vi "Motor controller.vi"() -> ()   [LabVIEW 2015]
uses:
  Motor controller/Signaller/Signaller.lvclass
  Motor controller/Motor/Motor.lvclass
  Motor controller/Automatic mode/Automatic Mode.lvclass
  Motor controller/Motor/AlphaStep One/AlphaStep One.lvclass
  Motor controller/Motor/Dummy Motor/Dummy Motor.lvclass
panel:
  in  "Home frequency 2":cluster{"Positive":dbl, "Negative":dbl}={"Positive"=140.18, "Negative"=140.45} {"Negative" format="%.3g"; "Positive" format="%.3g"}
  in  "Home frequency":cluster{"Positive":dbl, "Negative":dbl}={"Positive"=140.18, "Negative"=140.45} {"Negative" format="%.3g"; "Positive" format="%.3g"}
  in  "Negative seek bounds":cluster{"Minimum":dbl, "Maximum":dbl}={"Minimum"=140.35, "Maximum"=140.65} {"Maximum" format="%.3g"; "Minimum" format="%.3g"}
  in  "Positive seek bounds":cluster{"Minimum":dbl, "Maximum":dbl}={"Minimum"=140.0, "Maximum"=140.3} {"Maximum" format="%.3g"; "Minimum" format="%.3g"}
  in  "Debug mode":bool
  out "Grapher VI":refnum<vi>
  out "Simulation VI":refnum<vi>
  in  "0.01 GHz/step":bool
  in  "0.05 GHz/step":bool
  in  "0.03 GHz/step":bool
  in  "Reset everything":bool
  in  "Make up fit parameters":bool
  in  "Automatic velocity (rev/sec)":dbl=0.1 min=0.0 max=1.0
  in  "Reseek":bool
  in  "Automatic step size (rev)":dbl=0.01 min=0.0 max=1.0
  in  "Step size (GHz)":dbl min=0.0 max=1.0 step=0.001 format="%.3g"
  in  "Goto frequency":bool
  in  "Frequency to seek (GHz)":dbl format="%.3g"
  in  "Stop motor":bool
  in  "Move up":bool
  in  "Move down":bool
  in  "Velocity (rev/sec)":dbl min=0.0 max=1.0 step=0.001
  in  "Step size (rev)":dbl=0.01 min=0.0 max=5.0 step=0.001 format="%.3g"
  in  "Restore configuration from file":bool
  in  "Save configuration to file":bool
  in  "Refine fit parameters":bool
  out "Fit parameters":cluster{"Slope":dbl, "Intercept":dbl}
  in  "Calculate fit parameters":bool
  in  "Read position 2":bool
  in  "Read position 1":bool
  out "Position 2":dbl
  in  "Frequency 2":dbl=140.4 min=0.0 step=0.001 format="%.3g"
  out "Position 1":dbl
  in  "Frequency 1":dbl=140.0 min=0.0 step=0.001 format="%.3g"
  in  "Seek positive polarization":bool=TRUE
  in  "Launch simulation":bool
  out "Polarization":dbl
  out "Eventnum":i64
  out "Samples taken":i32
  out "Rate":dbl
  in  "Data input file":path
  in  "Automatic mode on/off":bool
  in  "Stop communication":bool
  in  "COM Port":refnum<visa-resource-name>
  out "Alarm":bool
  out "Alarm code":i32 format="0x%02x"
  out "Frequency (calculated, GHz)":dbl format="%.3g"
  out "Motor position (rev)":dbl format="%.3g"
  out "Motor time (sec)":dbl
  # "Advanced configuration"
  # "Step size presets"
  # "Manual motor control"
  # "Configuration backup/restore"
  # "The settings which are backed up by this method are: COM port, step size, frequency to seek, fit slope, fit intercept, automatic step size, automatic velocity, and data input file."
  # "Frequency calibration"
  # "Automatic control"
  # "Communication setup"
  # "Please wait after stopping the VI; it can take some time to shut down all the stuff running in the background, so please be patient."
  # "Motor alarm (error)"
  # "See motor manual, section \"Troubleshooting\" for explanation of alarm codes; fix the problem first and then restart this VI"
  # "Motor information"
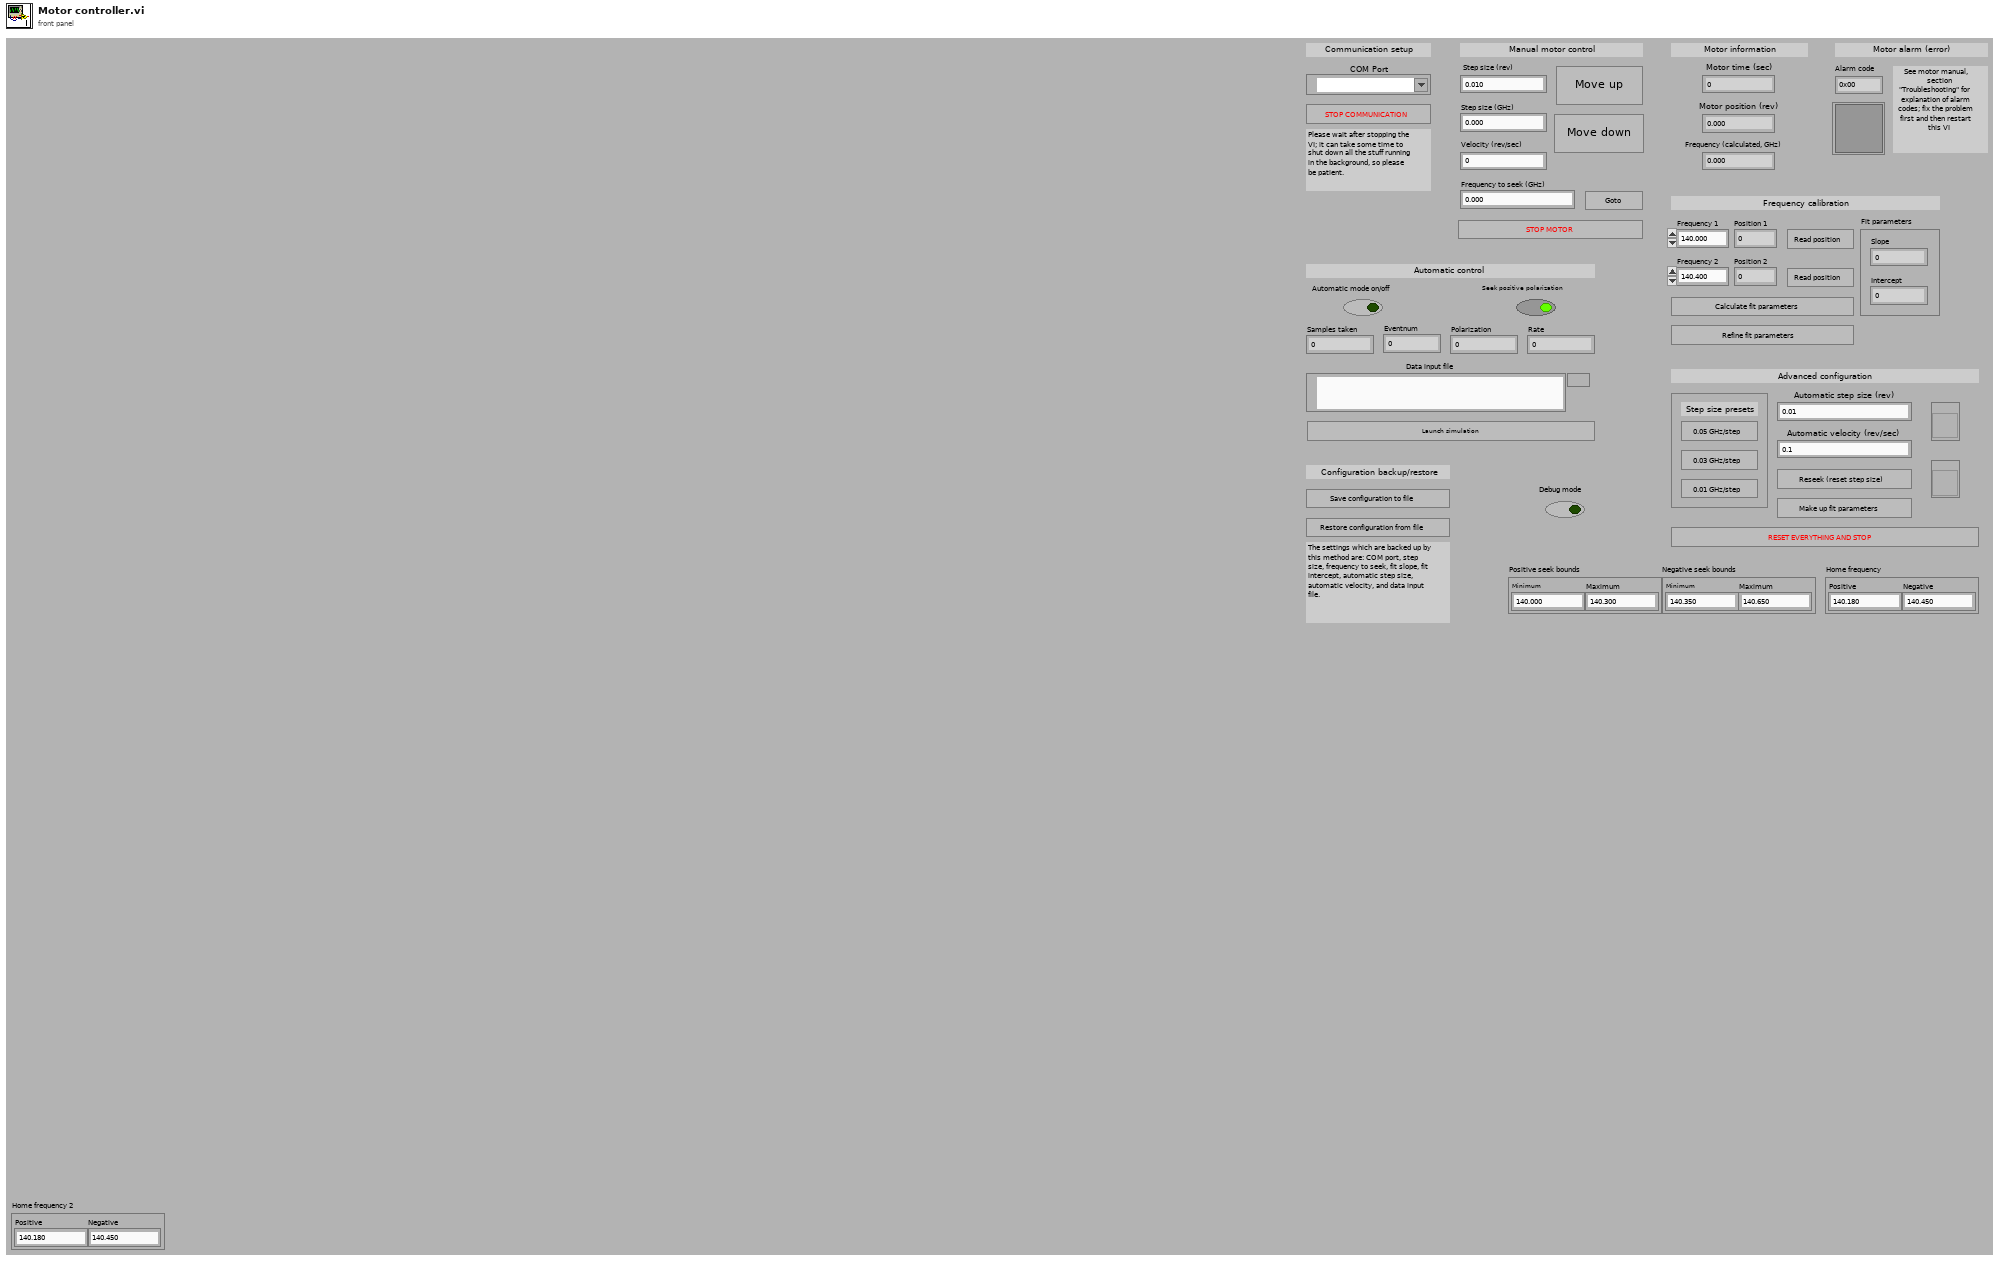
[diagram p1: front panel]
types:
  T1 = enum8{"Enabled", "Disabled", "Disabled and Grayed Out"}
  T2 = enum16{"open", "replace", "create", "open or create", "replace or create", "replace or create with confirmation"}
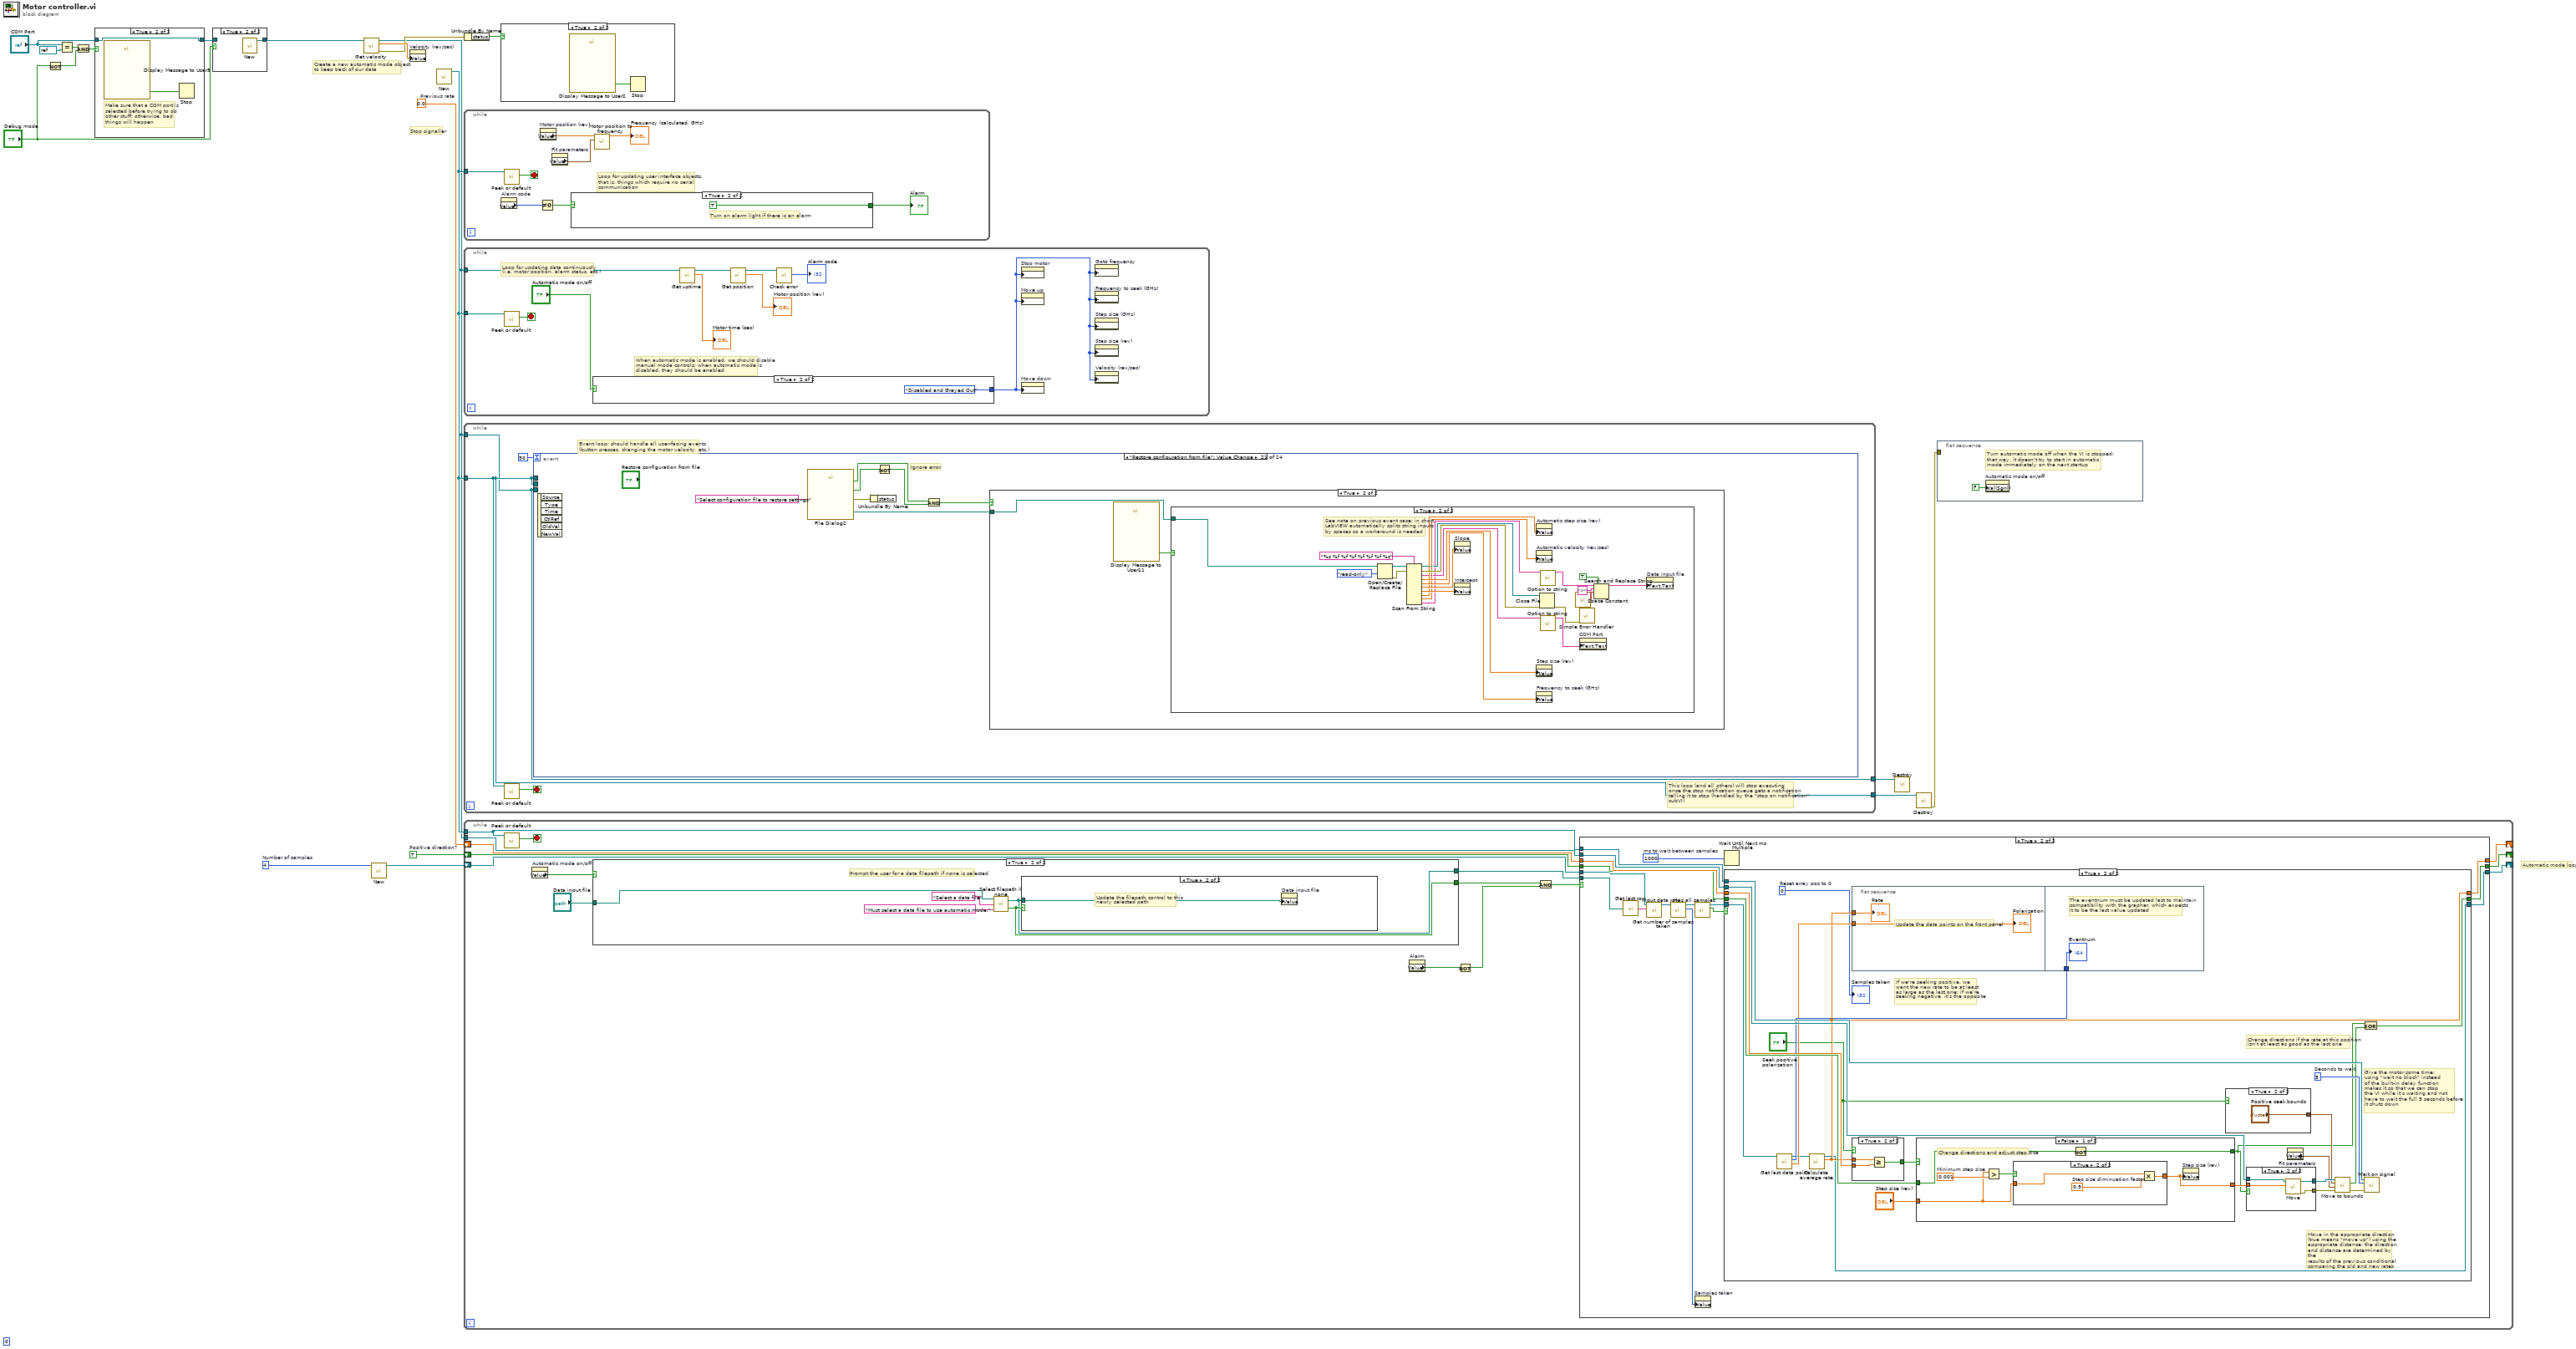
[diagram p0: block diagram]
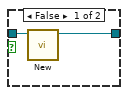
[diagram p2: hidden frame]
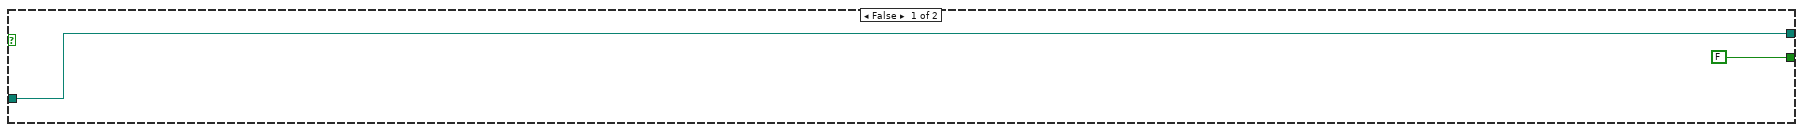
[diagram p5: hidden frame]
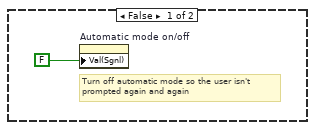
[diagram p6: hidden frame]
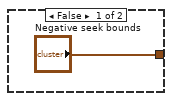
[diagram p9: hidden frame]
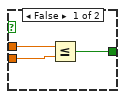
[diagram p10: hidden frame]
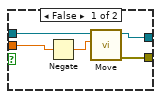
[diagram p11: hidden frame]
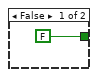
[diagram p14: hidden frame]
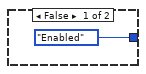
[diagram p15: hidden frame]
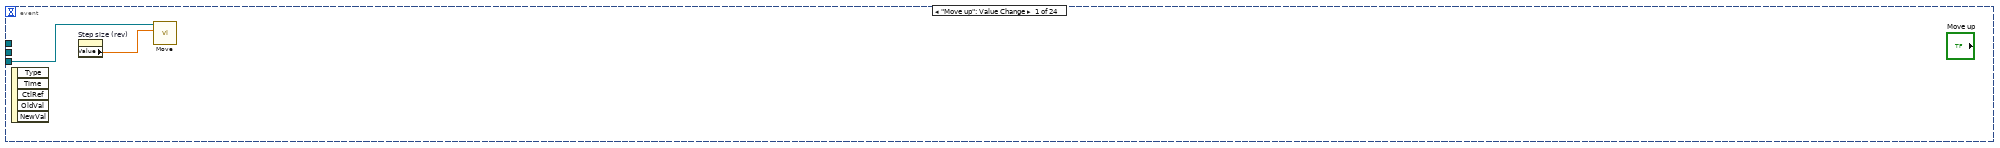
[diagram p16: hidden frame]
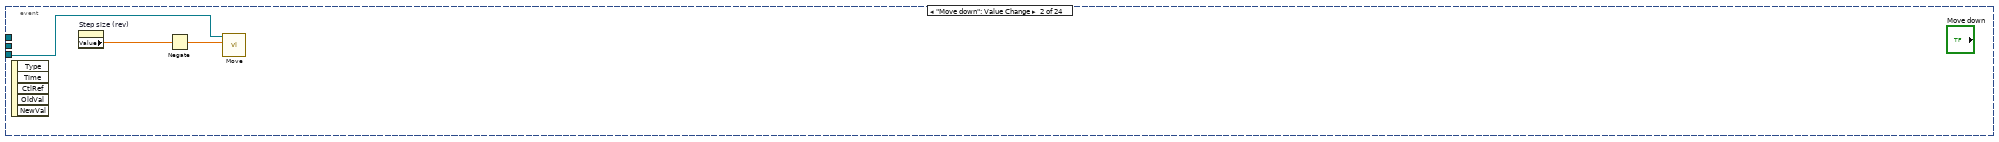
[diagram p17: hidden frame]
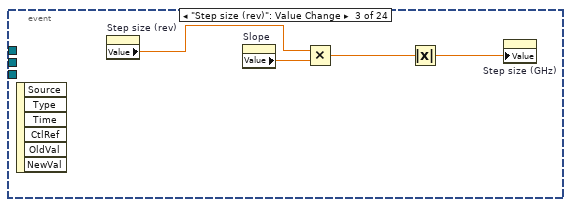
[diagram p18: hidden frame]
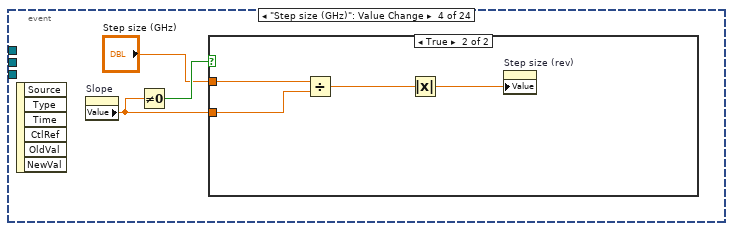
[diagram p19: hidden frame]
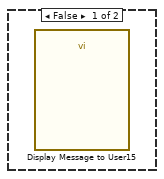
[diagram p20: hidden frame]
diagram:
  w14 = 4  # Number of samples
  w18 = TRUE  # Positive direction?
  w19 = 0.0  # Previous rate
  (unwired) i64 0
  # "Stop signaller"
  # "Create a new automatic mode object\nto keep track of our data"
  # "Automatic mode loop"
  n1 = Not(x="Debug mode") -> (.not. x?=w9:bool)
  n2 = Equal?(x="COM Port", y=refnum<visa-resource-name> refnum) -> (x = y?=w10:bool)
  n3 = And(x=w10, y=w9) -> (x .and. y?=w11:bool)
  n4 = case shown="True" w11 {
    tunnel: "COM Port" -> [w21 w22]
    tunnel: [w21 w22] -> w7
    frame False {
    }
    frame True {
      # "Make sure that a COM port is\nselected before trying to do\nother stuff; otherwise, bad\nthings will happen"
      n5 = call "Display Message to User5"() -> ("Got it, thanks"=w23:bool)  [unwired: 10 in, 1 out]
      n6 = Stop(stop? (T)=w23) -> ()
    }
  }
  n7 = case shown="True" "Debug mode" {
    tunnel: w7 -> [w25 _]
    tunnel: [w24 w26] -> w6
    frame False {
      n8 = call "New.vi"("VISA resource name"=w25) -> ("AlphaStep One out"=w24:refnum<class "AlphaStep One.lvclass">)  [unwired: 9 in, 1 out]
    }
    frame True {
      n9 = call "New.vi"() -> ("Dummy Motor out"=w26:refnum<class "Dummy Motor.lvclass">)  [unwired: 10 in, 1 out]
    }
  }
  n10 = call-dynamic "Get velocity.vi"("Motor in"=w6) -> ("error out"=w4:errorcluster, "Velocity (rev/sec)"=w5:dbl, "Motor out"=w3:refnum<class "Motor.lvclass">)  [unwired: 8 in]
  n11 = call "New.vi"("Number of samples (4)"=w14) -> ("Automatic Mode out"=w13:refnum<class "Automatic Mode.lvclass">)  [unwired: 9 in, 1 out]
  n12 = property on="Velocity (rev/sec)" class="DigNum (strict)"("Value"=w5) -> ()  [unwired: 2 in, 2 out]
  n13 = call "New.vi"() -> ("Signaller out"=w12:refnum<class "Signaller.lvclass">)  [unwired: 11 in]
  n14 = Unbundle By Name(w4) -> ("status"=w8:bool)
  n15 = while {
    tunnel: w12 -> [w30]
    stop <- w29 stop-if-true
    # "Loop for updating user interface objects,\nthat is, things which require no serial\ncommunication"
    n16 = property on="Alarm code" class="DigNum (strict)"() -> ("Value"=w28:i32)  [unwired: 2 in, 2 out]
    n17 = call "Peek or default.vi"("Signaller in"=w30) -> ("Has signal?"=w29:bool)  [unwired: 8 in, 2 out]
    n18 = property on="Motor position (rev)" class="DigNum (strict)"() -> ("Value"=w32:dbl)  [unwired: 2 in, 2 out]
    n19 = Not Equal To 0?(x=w28) -> (x != 0?=w27:bool)
    n20 = property on="Fit parameters" class="Clust (strict)"() -> ("Value"=w33:cluster{"Slope":dbl, "Intercept":dbl})  [unwired: 2 in, 2 out]
    n21 = case shown="True" w27 {
      tunnel: [FALSE TRUE] -> w34
      frame False {
      }
      frame True {
        # "Turn on alarm light if there is an alarm"
      }
    }
    "Alarm" <- w34
    n22 = call "Motor position to frequency.vi"("Fit parameters"=w33, "Motor position"=w32) -> ("Frequency"=→"Frequency (calculated, GHz)":dbl)  [unwired: 9 in]
  }
  n23 = while {
    tunnel: w3 -> [w42]
    tunnel: w12 -> [w45]
    stop <- w44 stop-if-true
    # "Loop for updating data continuously\n(i.e. motor position, alarm status, etc.)"
    # "When automatic mode is enabled, we should disable\nmanual mode controls; when automatic mode is\ndisabled, they should be enabled"
    n24 = call "Peek or default.vi"("Signaller in"=w45) -> ("Has signal?"=w44:bool)  [unwired: 8 in, 2 out]
    n25 = case shown="True" "Automatic mode on/off" {
      tunnel: [T1."Enabled" ("Disabled") T1."Disabled and Grayed Out" ("Disabled")] -> w43
      frame False {
      }
      frame True {
      }
    }
    n26 = call-dynamic "Get uptime.vi"("Motor in"=w42) -> ("Uptime (sec)"=→"Motor time (sec)":dbl, "Motor out"=w41:refnum<class "Motor.lvclass">)  [unwired: 8 in, 1 out]
    n27 = call-dynamic "Get position.vi"("Motor in"=w41) -> ("Position (rev)"=→"Motor position (rev)":dbl, "Motor out"=w38:refnum<class "Motor.lvclass">)  [unwired: 8 in, 1 out]
    n28 = call-dynamic "Check error.vi"("Motor in"=w38) -> ("Error code"=→"Alarm code":i32)  [unwired: 8 in, 2 out]
    n29 = property on="Stop motor" class="Bool"("DisabledEnum"=w43) -> ()  [unwired: 2 in, 2 out]
    n30 = property on="Move up" class="Bool"("DisabledEnum"=w43) -> ()  [unwired: 2 in, 2 out]
    n31 = property on="Move down" class="Bool"("DisabledEnum"=w43) -> ()  [unwired: 2 in, 2 out]
    n32 = property on="Goto frequency" class="Bool"("DisabledEnum"=w43) -> ()  [unwired: 2 in, 2 out]
    n33 = property on="Frequency to seek (GHz)" class="DigNum (strict)"("DisabledEnum"=w43) -> ()  [unwired: 2 in, 2 out]
    n34 = property on="Step size (GHz)" class="DigNum (strict)"("DisabledEnum"=w43) -> ()  [unwired: 2 in, 2 out]
    n35 = property on="Step size (rev)" class="DigNum (strict)"("DisabledEnum"=w43) -> ()  [unwired: 2 in, 2 out]
    n36 = property on="Velocity (rev/sec)" class="DigNum (strict)"("DisabledEnum"=w43) -> ()  [unwired: 2 in, 2 out]
  }
  n37 = while {
    tunnel: w3 -> [w49]
    tunnel: w12 -> [w50]
    tunnel: [w50] -> w20
    tunnel: [w49] -> w1
    stop <- w52 stop-if-true
    # "This loop (and all others) will stop executing\nonce the stop notification queue gets a notification\ntelling it to stop (handled by the \"stop on notification\"\nsubVI)"
    # "Event loop; should handle all user-facing events\n(button presses, changing the motor velocity, etc.)"
    n38 = call "Peek or default.vi"("Signaller in"=w50) -> ("Has signal?"=w52:bool)  [unwired: 8 in, 2 out]
    n39 = event shown="[20] \"Restore configuration from file\": Value Change" {
      selector: _ -> [_ _ _ _ _ _ _ _ _ _ _ _ _ _ _ _ _ _ _ _ _ _ _ _]
      dyn-events: _ -> [_ _ _ _ _ _ _ _ _ _ _ _ _ _ _ _ _ _ _ _ _ _ _ _]
      timeout: 50 -> [_ _ _ _ _ _ _ _ _ _ _ _ _ _ _ _ _ _ _ _ _ _ _ _]
      tunnel: w49 -> [w53 w55 _ _ w70 w72 w92 _ _ _ _ _ _ w173 w204 _ _ _ _ _ _ _ w313 _]
      tunnel: w50 -> [_ _ _ _ _ _ _ _ _ _ _ w153 _ _ _ _ _ _ _ _ _ w308 w316 _]
      tunnel: w50 -> [_ _ _ _ _ _ _ _ _ _ _ _ _ w174 _ _ _ _ _ _ _ _ _ _]
      event "Move up": Value Change {
        n40 = event-data() -> ()  [unwired: 1 in, 5 out]
        n41 = property on="Step size (rev)" class="DigNum (strict)"() -> ("Value"=w54:dbl)  [unwired: 2 in, 2 out]
        n42 = call-dynamic "Move.vi"("Amount (rev)"=w54, "Motor in"=w53) -> ()  [unwired: 8 in, 2 out]
      }
      event "Move down": Value Change {
        n43 = event-data() -> ()  [unwired: 1 in, 5 out]
        n44 = property on="Step size (rev)" class="DigNum (strict)"() -> ("Value"=w57:dbl)  [unwired: 2 in, 2 out]
        n45 = Negate(x=w57) -> (-x=w56:dbl)
        n46 = call-dynamic "Move.vi"("Amount (rev)"=w56, "Motor in"=w55) -> ()  [unwired: 8 in, 2 out]
      }
      event "Step size (rev)": Value Change {
        n47 = event-data() -> ()  [unwired: 1 in, 6 out]
        n48 = property on="Step size (rev)" class="DigNum (strict)"() -> ("Value"=w61:dbl)  [unwired: 2 in, 2 out]
        n49 = property on="Slope" class="DigNum (strict)"() -> ("Value"=w60:dbl)  [unwired: 2 in, 2 out]
        n50 = Multiply(x=w61, y=w60) -> (x*y=w59:dbl)
        n51 = Absolute Value(x=w59) -> (abs(x)=w58:dbl)
        n52 = property on="Step size (GHz)" class="DigNum (strict)"("Value"=w58) -> ()  [unwired: 2 in, 2 out]
      }
      event "Step size (GHz)": Value Change {
        n53 = event-data() -> ()  [unwired: 1 in, 6 out]
        n54 = property on="Slope" class="DigNum (strict)"() -> ("Value"=w62:dbl)  [unwired: 2 in, 2 out]
        n55 = Not Equal To 0?(x=w62) -> (x != 0?=w64:bool)
        n56 = case shown="True" w64 {
          tunnel: "Step size (GHz)" -> [_ w68]
          tunnel: w62 -> [_ w67]
          frame False {
            n57 = call "Display Message to User15"() -> ()  [unwired: 10 in, 2 out]
          }
          frame True {
            n58 = Divide(x=w68, y=w67) -> (x/y=w66:dbl)
            n59 = Absolute Value(x=w66) -> (abs(x)=w65:dbl)
            n60 = property on="Step size (rev)" class="DigNum (strict)"("Value"=w65) -> ()  [unwired: 2 in, 2 out]
          }
        }
      }
      event "Velocity (rev/sec)": Value Change {
        n61 = event-data() -> ()  [unwired: 1 in, 5 out]
        n62 = call-dynamic "Set velocity.vi"("Velocity (rev/sec)"="Velocity (rev/sec)", "Motor in"=w70) -> ()  [unwired: 8 in, 2 out]
      }
      event "Goto frequency": Value Change {
        n63 = event-data() -> ()  [unwired: 1 in, 5 out]
        n64 = property on="Fit parameters" class="Clust (strict)"() -> ("Value"=w71:cluster{"Slope":dbl, "Intercept":dbl})  [unwired: 2 in, 2 out]
        n65 = Unbundle By Name(w71) -> ("Slope"=w73:dbl)
        n66 = Equal To 0?(x=w73) -> (x = 0?=w74:bool)
        n67 = case shown="False" w74 {
          tunnel: w72 -> [w82 _]
          tunnel: w71 -> [w75 _]
          frame False {
            # "Calculate corresponding motor position and go there"
            n68 = call "Frequency to motor position.vi"("Fit parameters"=w75, "Frequency"="Frequency to seek (GHz)") -> ("Motor position"=w84:dbl)  [unwired: 9 in]
            n69 = property on="Motor position (rev)" class="DigNum (strict)"() -> ("Value"=w83:dbl)  [unwired: 2 in, 2 out]
            n70 = Subtract(x=w84, y=w83) -> (x-y=w80:dbl)
            n71 = Absolute Value(x=w80) -> (abs(x)=w79:dbl)
            n72 = Less?(x=w79, y=1.0) -> (x < y?=w76:bool)
            n73 = case shown="False" w76 {
              selector: w76 -> [_ w89]
              tunnel: [w85 w89] -> w77
              frame False {
                n74 = Two Button Dialog(message="The frequency you are attempting to go to is very far from the current position; you may run into problems. Are you sure you want to continue?", 1:"No" ("F button name (\"Cancel\")"), 2:"Yes" ("T button name (\"OK\")")) -> (T button?=w85:bool)
              }
              frame True {
              }
            }
            n75 = case shown="True" w77 {
              tunnel: w82 -> [_ w90]
              tunnel: w80 -> [_ w91]
              frame False {
              }
              frame True {
                n76 = call-dynamic "Move.vi"("Amount (rev)"=w91, "Motor in"=w90) -> ()  [unwired: 8 in, 2 out]
              }
            }
          }
          frame True {
            n77 = call "Display Message to User"() -> ()  [unwired: 10 in, 2 out]
          }
        }
      }
      event "Stop motor": Value Change {
        n78 = event-data() -> ()  [unwired: 1 in, 5 out]
        n79 = call-dynamic "Stop.vi"("Motor in"=w92) -> ()  [unwired: 9 in, 2 out]
      }
      event "Read position 1": Value Change {
        n80 = event-data() -> ()  [unwired: 1 in, 5 out]
        n81 = property on="Motor position (rev)" class="DigNum (strict)"() -> ("Value"=→"Position 1":dbl)  [unwired: 2 in, 2 out]
      }
      event "Read position 2": Value Change {
        n82 = event-data() -> ()  [unwired: 1 in, 5 out]
        n83 = property on="Motor position (rev)" class="DigNum (strict)"() -> ("Value"=→"Position 2":dbl)  [unwired: 2 in, 2 out]
      }
      event "Calculate fit parameters": Value Change {
        n84 = event-data() -> ()  [unwired: 1 in, 5 out]
        n85 = property on="Position 1" class="DigNum (strict)"() -> ("Value"=w99:dbl)  [unwired: 2 in, 2 out]
        n86 = property on="Position 2" class="DigNum (strict)"() -> ("Value"=w98:dbl)  [unwired: 2 in, 2 out]
        n87 = property on="Calculate fit parameters" class="Bool (strict)"("Value"=FALSE ("Calculate fit parameters")) -> ()  [unwired: 2 in, 2 out]
        n88 = Equal?(x=w99, y=w98) -> (x = y?=w101:bool)
        n89 = Equal?(x="Frequency 1", y="Frequency 2") -> (x = y?=w100:bool)
        n90 = Or(x=w101, y=w100) -> (x .or. y?=w95:bool)
        n91 = case shown="False" w95 {
          tunnel: w99 -> [w110 _]
          tunnel: w98 -> [w109 _]
          tunnel: "Frequency 1" -> [w108 _]
          tunnel: "Frequency 2" -> [w107 _]
          frame False {
            # "Calculate slope and intercept"
            # "The automatic step size should be around 0.02GHz\ninitially, to get a good seek"
            n92 = call "Calculate fit parameters.vi"("Frequency 2"=w107, "Frequency 1"=w108, "Position 2"=w109, "Position 1"=w110) -> ("Intercept"=w111:dbl, "Slope"=w105:dbl)
            n93 = property on="Fit parameters" class="Clust (strict)"() -> ("Value"=w113:cluster{"Slope":dbl, "Intercept":dbl})  [unwired: 2 in, 2 out]
            n94 = Divide(x=0.02, y=w105) -> (x/y=w104:dbl)
            n95 = Bundle By Name(cluster=w113, "Slope"=w105, "Intercept"=w111) -> (→"Fit parameters":cluster{"Slope":dbl, "Intercept":dbl})
            n96 = Absolute Value(x=w104) -> (abs(x)=w103:dbl)
            n97 = property on="Automatic step size (rev)" class="DigNum (strict)"("Value"=w103) -> ()  [unwired: 2 in, 2 out]
          }
          frame True {
            # "Warn the user about trying to calculate/refine\nfit parameters with invalid inputs (fit function\nMUST be bijective; i.e. slope must not be 0\nor infinity)"
            n98 = call "Display Message to User6"() -> ()  [unwired: 10 in, 2 out]
          }
        }
      }
      event "Refine fit parameters": Value Change {
        n99 = event-data() -> ()  [unwired: 1 in, 6 out]
        n100 = property on="Fit parameters" class="Clust (strict)"() -> ("Value"=w119:cluster{"Slope":dbl, "Intercept":dbl})  [unwired: 2 in, 2 out]
        n101 = Unbundle By Name(w119) -> ("Slope"=w115:dbl, "Intercept"=w114:dbl)
        n102 = Equal To 0?(x=w115) -> (x = 0?=w117:bool)
        n103 = Equal To 0?(x=w114) -> (x = 0?=w116:bool)
        n104 = And(x=w116, y=w117) -> (x .and. y?=w118:bool)
        n105 = property on="Frequency 1" class="DigNum (strict)"() -> ("Value"=w123:dbl)  [unwired: 2 in, 2 out]
        n106 = property on="Frequency 2" class="DigNum (strict)"() -> ("Value"=w122:dbl)  [unwired: 2 in, 2 out]
        n107 = property on="Position 1" class="DigNum (strict)"() -> ("Value"=w121:dbl)  [unwired: 2 in, 2 out]
        n108 = property on="Position 2" class="DigNum (strict)"() -> ("Value"=w120:dbl)  [unwired: 2 in, 2 out]
        n109 = case shown="False" w118 {
          tunnel: w123 -> [w125 _]
          tunnel: w122 -> [w124 _]
          tunnel: w121 -> [w130 _]
          tunnel: w120 -> [w129 _]
          tunnel: w115 -> [w133 _]
          tunnel: w114 -> [w132 _]
          tunnel: w119 -> [w131 _]
          frame False {
            n110 = Equal?(x=w130, y=w129) -> (x = y?=w128:bool)
            n111 = Equal?(x=w125, y=w124) -> (x = y?=w127:bool)
            n112 = Or(x=w128, y=w127) -> (x .or. y?=w126:bool)
            n113 = case shown="False" w126 {
              tunnel: w125 -> [w152 _]
              tunnel: w124 -> [w151 _]
              tunnel: w130 -> [w150 _]
              tunnel: w129 -> [w149 _]
              tunnel: w133 -> [w147 _]
              tunnel: w132 -> [w145 _]
              tunnel: w131 -> [w139 _]
              frame False {
                # "Update automatic step size as well,\nas with the \"calculate fit parameters\"\naction"
                # "Average new slope and intercept with\nold ones, to get better approximation"
                n114 = call "Calculate fit parameters.vi"("Frequency 2"=w151, "Frequency 1"=w152, "Position 2"=w149, "Position 1"=w150) -> ("Intercept"=w146:dbl, "Slope"=w148:dbl)
                n115 = Add(x=w148, y=w147) -> (x+y=w144:dbl)
                n116 = Add(x=w146, y=w145) -> (x+y=w143:dbl)
                n117 = Divide(x=w144, y=2.0) -> (x/y=w136:dbl)
                n118 = Divide(x=w143, y=2.0) -> (x/y=w138:dbl)
                n119 = Bundle By Name(cluster=w139, "Slope"=w136, "Intercept"=w138) -> (w140:cluster{"Slope":dbl, "Intercept":dbl})
                n120 = Divide(x=0.02, y=w136) -> (x/y=w135:dbl)
                n121 = property on="Fit parameters" class="Clust (strict)"("Value"=w140) -> ()  [unwired: 2 in, 2 out]
                n122 = Absolute Value(x=w135) -> (abs(x)=w134:dbl)
                n123 = property on="Automatic step size (rev)" class="DigNum (strict)"("Value"=w134) -> ()  [unwired: 2 in, 2 out]
              }
              frame True {
                # "Warn the user about trying to calculate/refine\nfit parameters with invalid inputs (fit function\nMUST be bijective; i.e. slope must not be 0\nor infinity)"
                n124 = call "Display Message to User7"() -> ()  [unwired: 10 in, 2 out]
              }
            }
          }
          frame True {
            # "Warn the user about refining fit parameters\nwithout calculating initial parameters first"
            n125 = call "Display Message to User4"() -> ()  [unwired: 10 in, 2 out]
          }
        }
      }
      event "Launch simulation": Value Change {
        # "Tell the simulation notifier to launch the simulation"
        n126 = event-data() -> ()  [unwired: 1 in, 5 out]
        n127 = property on="Fit parameters" class="Clust (strict)"() -> ("Value"=w156:cluster{"Slope":dbl, "Intercept":dbl})  [unwired: 2 in, 2 out]
        n128 = Unbundle By Name(w156) -> ("Slope"=w155:dbl)
        n129 = Equal To 0?(x=w155) -> (x = 0?=w154:bool)
        n130 = case shown="False" w154 {
          tunnel: w153 -> [w161 _]
          frame False {
            n131 = property on="Simulation VI" class="VIRef (strict)"() -> ("Value"=w159:refnum<vi>)  [unwired: 2 in, 2 out]
            n132 = Not A Number/Path/Refnum?(number/path/refnum=w159) -> (NaN/Path/Refnum?=w160:bool)
            n133 = case shown="True" w160 {
              tunnel: w161 -> [_ w165]
              tunnel: [w162 w164] -> w158
              tunnel: w159 -> [w162 _]
              frame False {
              }
              frame True {
                n134 = vi-ref "Simulation.vi"() -> (w170:refnum<vi>)
                n135 = property class="VI Interface Type 1"(reference=w170) -> ("Name"=w169:string)  [unwired: 1 in, 2 out]
                n136 = control-ref of="Frequency (calculated, GHz)"() -> (w166:refnum<vi>)
                n137 = Open VI Reference(type specifier VI Refnum (for type only)=w170, vi path=w169, options=128) -> (vi reference=w168:refnum<vi>)  [unwired: 3 in, 1 out]
                n138 = control-ref of="Data input file"() -> (w167:refnum<vi>)
                n139 = call-by-ref "Start Asynchronous Call"(reference=w168, "Stop signaller"=w165, "Frequency refnum"=w166, "Data input file refnum"=w167) -> (reference out=w164:refnum<vi>)  [unwired: 2 in, 1 out]
              }
            }
            n140 = invoke class="VI Interface Type 0" method="FP.Open"(reference=w158) -> (reference out=→"Simulation VI":refnum<vi>)  [unwired: 4 in, 4 out]
          }
          frame True {
            n141 = call "Display Message to User3"() -> ()  [unwired: 10 in, 2 out]
          }
        }
      }
      event "Reseek": Value Change {
        # "Change step size back to the default (initial) automatic step size"
        n142 = event-data() -> ()  [unwired: 1 in, 5 out]
        n143 = property on="Automatic mode on/off" class="Bool (strict)"() -> ("Value"=w171:bool)  [unwired: 2 in, 2 out]
        n144 = case shown="True" w171 {
          frame False {
          }
          frame True {
            n145 = property on="Automatic step size (rev)" class="DigNum (strict)"() -> ("Value"=w172:dbl)  [unwired: 2 in, 2 out]
            n146 = property on="Step size (rev)" class="DigNum (strict)"("Val(Sgnl)"=w172) -> ()  [unwired: 2 in, 2 out]
          }
        }
      }
      event "Automatic mode on/off": Value Change {
        # "When automatic mode is first enabled,\nchoose the initial step size and start\ngrapher subvi"
        n147 = event-data() -> ()  [unwired: 1 in, 5 out]
        n148 = property on="Automatic mode on/off" class="Bool (strict)"() -> ("Value"=w175:bool)  [unwired: 2 in, 2 out]
        n149 = case shown="True" w175 {
          tunnel: w174 -> [_ w186]
          tunnel: w173 -> [_ w179]
          frame False {
          }
          frame True {
            # "Move to home position"
            n150 = property on="Grapher VI" class="VIRef (strict)"() -> ("Value"=w182:refnum<vi>)  [unwired: 2 in, 2 out]
            n151 = Not A Number/Path/Refnum?(number/path/refnum=w182) -> (NaN/Path/Refnum?=w183:bool)
            n152 = property on="Seek positive polarization" class="Bool (strict)"() -> ("Value"=w181:bool)  [unwired: 2 in, 2 out]
            n153 = case shown="True" w183 {
              tunnel: w186 -> [_ w195]
              tunnel: [w193 w194] -> w185
              tunnel: w182 -> [w193 _]
              frame False {
              }
              frame True {
                n154 = vi-ref "Grapher.vi"() -> (w203:refnum<vi>)
                n155 = property class="VI Interface Type 0"(reference=w203) -> ("Name"=w202:string)  [unwired: 1 in, 2 out]
                n156 = Open VI Reference(type specifier VI Refnum (for type only)=w203, vi path=w202, options=128) -> (vi reference=w200:refnum<vi>)  [unwired: 3 in, 1 out]
                n157 = control-ref of="Frequency (calculated, GHz)"() -> (w198:refnum<vi>)
                n158 = control-ref of="Polarization"() -> (w197:refnum<vi>)
                n159 = control-ref of="Eventnum"() -> (w199:refnum<vi>)
                n160 = control-ref of="Rate"() -> (w196:refnum<vi>)
                n161 = call-by-ref "Start Asynchronous Call"(reference=w200, "Eventnum refnum"=w199, "Frequency refnum"=w198, "Stop signaller"=w195, "Polarization refnum"=w197, "Rate refnum"=w196) -> (reference out=w194:refnum<vi>)  [unwired: 12 in, 1 out]
              }
            }
            n162 = case shown="False" w181 {
              tunnel: "Home frequency" -> [w190 w192]
              tunnel: [w189 w191] -> w178
              frame False {
                n163 = Unbundle By Name(w190) -> ("Negative"=w189:dbl)
              }
              frame True {
                n164 = Unbundle By Name(w192) -> ("Positive"=w191:dbl)
              }
            }
            n165 = property on="Step size (rev)" class="DigNum (strict)"("Val(Sgnl)"="Automatic step size (rev)") -> ()  [unwired: 2 in, 2 out]
            n166 = property on="Velocity (rev/sec)" class="DigNum (strict)"("Val(Sgnl)"="Automatic velocity (rev/sec)") -> ()  [unwired: 2 in, 2 out]
            n167 = property on="Fit parameters" class="Clust (strict)"() -> ("Value"=w176:cluster{"Slope":dbl, "Intercept":dbl})  [unwired: 2 in, 2 out]
            n168 = call "Frequency to motor position.vi"("Fit parameters"=w176, "Frequency"=w178) -> ("Motor position"=w177:dbl)  [unwired: 9 in]
            n169 = call-dynamic "Move to position.vi"("Position"=w177, "Motor in"=w179) -> ()  [unwired: 8 in, 2 out]
            n170 = invoke class="VI Interface Type 1" method="FP.Open"(reference=w185) -> (reference out=→"Grapher VI":refnum<vi>)  [unwired: 4 in, 4 out]
          }
        }
      }
      event "Seek positive polarization": Value Change {
        # "Move to home position"
        n171 = event-data() -> ()  [unwired: 1 in, 6 out]
        n172 = property on="Seek positive polarization" class="Bool (strict)"() -> ("Value"=w206:bool)  [unwired: 2 in, 2 out]
        n173 = case shown="False" w206 {
          tunnel: "Home frequency 2" -> [w211 w213]
          tunnel: [w210 w212] -> w208
          frame False {
            n174 = Unbundle By Name(w211) -> ("Negative"=w210:dbl)
          }
          frame True {
            n175 = Unbundle By Name(w213) -> ("Positive"=w212:dbl)
          }
        }
        n176 = property on="Fit parameters" class="Clust (strict)"() -> ("Value"=w205:cluster{"Slope":dbl, "Intercept":dbl})  [unwired: 2 in, 2 out]
        n177 = call "Frequency to motor position.vi"("Fit parameters"=w205, "Frequency"=w208) -> ("Motor position"=w207:dbl)  [unwired: 9 in]
        n178 = call-dynamic "Move to position.vi"("Position"=w207, "Motor in"=w204) -> ()  [unwired: 8 in, 2 out]
      }
      event "0.05 GHz/step": Value Change {
        n179 = event-data() -> ()  [unwired: 1 in, 6 out]
        n180 = property on="Slope" class="DigNum (strict)"() -> ("Value"=w214:dbl)  [unwired: 2 in, 2 out]
        n181 = Not Equal To 0?(x=w214) -> (x != 0?=w215:bool)
        n182 = case shown="True" w215 {
          tunnel: w214 -> [_ w218]
          frame False {
            n183 = call "Display Message to User12"() -> ()  [unwired: 10 in, 2 out]
          }
          frame True {
            n184 = Divide(x=0.05, y=w218) -> (x/y=w217:dbl)
            n185 = Absolute Value(x=w217) -> (abs(x)=w216:dbl)
            n186 = property on="Automatic step size (rev)" class="DigNum (strict)"("Value"=w216) -> ()  [unwired: 2 in, 2 out]
          }
        }
      }
      event "0.03 GHz/step": Value Change {
        n187 = event-data() -> ()  [unwired: 1 in, 6 out]
        n188 = property on="Slope" class="DigNum (strict)"() -> ("Value"=w220:dbl)  [unwired: 2 in, 2 out]
        n189 = Not Equal To 0?(x=w220) -> (x != 0?=w221:bool)
        n190 = case shown="True" w221 {
          tunnel: w220 -> [_ w224]
          frame False {
            n191 = call "Display Message to User13"() -> ()  [unwired: 10 in, 2 out]
          }
          frame True {
            n192 = Divide(x=0.03, y=w224) -> (x/y=w223:dbl)
            n193 = Absolute Value(x=w223) -> (abs(x)=w222:dbl)
            n194 = property on="Automatic step size (rev)" class="DigNum (strict)"("Value"=w222) -> ()  [unwired: 2 in, 2 out]
          }
        }
      }
      event "0.01 GHz/step": Value Change {
        n195 = event-data() -> ()  [unwired: 1 in, 6 out]
        n196 = property on="Slope" class="DigNum (strict)"() -> ("Value"=w226:dbl)  [unwired: 2 in, 2 out]
        n197 = Not Equal To 0?(x=w226) -> (x != 0?=w227:bool)
        n198 = case shown="True" w227 {
          tunnel: w226 -> [_ w230]
          frame False {
            n199 = call "Display Message to User14"() -> ()  [unwired: 10 in, 2 out]
          }
          frame True {
            n200 = Divide(x=0.01, y=w230) -> (x/y=w229:dbl)
            n201 = Absolute Value(x=w229) -> (abs(x)=w228:dbl)
            n202 = property on="Automatic step size (rev)" class="DigNum (strict)"("Value"=w228) -> ()  [unwired: 2 in, 2 out]
          }
        }
      }
      event "Make up fit parameters": Value Change {
        # "Make up some fit parameters (no physical meaning)\nfor quick testing of automatic mode"
        n203 = event-data() -> ()  [unwired: 1 in, 5 out]
        n204 = flat-sequence {
          frame #0 {
            n205 = property on="Frequency 1" class="DigNum (strict)"("Value"=140.1 ("Frequency 1")) -> ()  [unwired: 2 in, 2 out]
            n206 = property on="Frequency 2" class="DigNum (strict)"("Value"=140.15 ("Frequency 2")) -> ()  [unwired: 2 in, 2 out]
            n207 = property on="Motor position (rev)" class="DigNum (strict)"() -> ("Value"=w236:dbl)  [unwired: 2 in, 2 out]
            n208 = property on="Step size (rev)" class="DigNum (strict)"() -> ("Value"=w234:dbl)  [unwired: 2 in, 2 out]
            n209 = property on="Position 2" class="DigNum (strict)"("Value"=w236) -> ()  [unwired: 2 in, 2 out]
            n210 = Subtract(x=w236, y=w234) -> (x-y=w235:dbl)
            n211 = property on="Position 1" class="DigNum (strict)"("Value"=w235) -> ()  [unwired: 2 in, 2 out]
          }
          frame #1 {
            n212 = property on="Calculate fit parameters" class="Bool (strict)"("Val(Sgnl)"=TRUE ("Value (Signaling)")) -> ()  [unwired: 2 in, 2 out]
          }
        }
      }
      event "Save configuration to file": Value Change {
        # "Ignore error"
        n213 = event-data() -> ()  [unwired: 1 in, 6 out]
        n214 = call "File Dialog"("prompt"="Select file to store configuration", "default name"="controller_settings.txt") -> ("selected path"=w243:path, "exists"=w244:bool, "cancelled"=w241:bool, "error out"=w239:errorcluster)  [unwired: 10 in]
        n215 = Unbundle By Name(w239) -> ()  [unwired: 1 out]
        n216 = Not A Number/Path/Refnum?(number/path/refnum=w243) -> (NaN/Path/Refnum?=w242:bool)
        n217 = Or(x=w242, y=w241) -> (x .or. y?=w240:bool)
        n218 = case shown="False" w240 {
          tunnel: w244 -> [w248 _]
          tunnel: w243 -> [w246 _]
          frame False {
            n219 = case shown="True" w248 {
              tunnel: [TRUE ("Yes") w272] -> w247
              frame False {
              }
              frame True {
                n220 = call "Display Message to User9"() -> ("Yes"=w272:bool)  [unwired: 10 in, 1 out]
              }
            }
            n221 = case shown="True" w247 {
              tunnel: w246 -> [_ w270]
              frame False {
              }
              frame True {
                # "Labview won't be able to scan in a string with spaces :(\n> is an illegal filepath character in Windows,\nso this will never cause problems"
                # "Save any important configuration"
                n222 = property on="Data input file" class="Path"() -> ("Text.Text"=w255:string)  [unwired: 2 in, 2 out]
                n223 = call <vilib>:"Space Constant.vi"() -> ("String"=w254:string)
                n224 = Search and Replace String(replace all?=TRUE ("replace all? (F)"), input string=w255, search string=w254, replace string=">" ("replace string (\"\")")) -> (result string=w250:string)  [unwired: 4 in, 3 out]
                n225 = property on="COM Port" class="VISAName"() -> ("Text.Text"=w252:string)  [unwired: 2 in, 2 out]
                n226 = property on="Automatic velocity (rev/sec)" class="DigNum (strict)"() -> ("Value"=w258:dbl)  [unwired: 2 in, 2 out]
                n227 = property on="Automatic step size (rev)" class="DigNum (strict)"() -> ("Value"=w259:dbl)  [unwired: 2 in, 2 out]
                n228 = property on="Frequency to seek (GHz)" class="DigNum (strict)"() -> ("Value"=w262:dbl)  [unwired: 2 in, 2 out]
                n229 = property on="Step size (rev)" class="DigNum (strict)"() -> ("Value"=w263:dbl)  [unwired: 2 in, 2 out]
                n230 = Open/Create/Replace File(file path (use dialog)=w270, operation (0:open)=T2."replace or create", access (0:read/write)=enum16{"read/write", "read-only", "write-only"}."write-only") -> (refnum out=w268:refnum<file>, error out=w267:errorcluster)  [unwired: 3 in, 1 out]
                n231 = call "String to option.vi"("String in"=w252) -> ("String out"=w251:string)  [unwired: 10 in]
                n232 = call "String to option.vi"("String in"=w250) -> ("String out"=w249:string)  [unwired: 10 in]
                n233 = property on="Intercept" class="DigNum (strict)"() -> ("Value"=w260:dbl)  [unwired: 2 in, 2 out]
                n234 = property on="Slope" class="DigNum (strict)"() -> ("Value"=w261:dbl)  [unwired: 2 in, 2 out]
                n235 = Format Into String(initial string=w268, error in=w267, w251, w263, w262, w261, w260, w259, w258, w249) -> (resulting string=w265:refnum<file>, error out=w266:errorcluster)  [unwired: 1 in]
                n236 = Close File(refnum=w265, error in=w266) -> (error out=w264:errorcluster)  [unwired: 1 out]
                n237 = call <vilib>:"Simple Error Handler.vi"("error in (no error)"=w264) -> ()  [unwired: 4 in, 5 out]
              }
            }
          }
          frame True {
            n238 = call "Display Message to User8"() -> ()  [unwired: 10 in, 2 out]
          }
        }
      }
      event "Restore configuration from file": Value Change {
        # "Ignore error"
        n239 = event-data() -> ()  [unwired: 1 in, 6 out]
        n240 = call "File Dialog2"("prompt"="Select configuration file to restore settings") -> ("selected path"=w278:path, "exists"=w277:bool, "cancelled"=w275:bool, "error out"=w273:errorcluster)  [unwired: 11 in]
        n241 = Unbundle By Name(w273) -> ()  [unwired: 1 out]
        n242 = Not(x=w275) -> (.not. x?=w274:bool)
        n243 = And(x=w277, y=w274) -> (x .and. y?=w276:bool)
        n244 = case shown="True" w276 {
          tunnel: w278 -> [_ w280]
          frame False {
            n245 = call "Display Message to User10"() -> ()  [unwired: 10 in, 2 out]
          }
          frame True {
            n246 = call "Display Message to User11"() -> ("Yes"=w281:bool)  [unwired: 10 in, 1 out]
            n247 = case shown="True" w281 {
              tunnel: w280 -> [_ w303]
              frame False {
              }
              frame True {
                # "See note on previous event case; in short,\nLabVIEW automatically splits string inputs\nby spaces so a workaround is needed"
                n248 = Open/Create/Replace File(file path (use dialog)=w303, access (0:read/write)=enum16{"read/write", "read-only", "write-only"}."read-only") -> (refnum out=w292:refnum<file>, error out=w301:errorcluster)  [unwired: 4 in, 1 out]
                n249 = Scan From String("%s %f %f %f %f %f %f %s" ("format string"), w292, w301) -> (w291:refnum<file>, w300:errorcluster, output 1=w285:string, output 2=w298:dbl, output 3=w297:dbl, output 4=w296:dbl, output 5=w295:dbl, output 6=w294:dbl, output 7=w293:dbl, output 8=w283:string)  [unwired: 8 in]
                n250 = property on="Slope" class="DigNum (strict)"("Value"=w296) -> ()  [unwired: 2 in, 2 out]
                n251 = property on="Intercept" class="DigNum (strict)"("Value"=w295) -> ()  [unwired: 2 in, 2 out]
                n252 = property on="Automatic step size (rev)" class="DigNum (strict)"("Value"=w294) -> ()  [unwired: 2 in, 2 out]
                n253 = property on="Automatic velocity (rev/sec)" class="DigNum (strict)"("Value"=w293) -> ()  [unwired: 2 in, 2 out]
                n254 = property on="Step size (rev)" class="DigNum (strict)"("Value"=w298) -> ()  [unwired: 2 in, 2 out]
                n255 = property on="Frequency to seek (GHz)" class="DigNum (strict)"("Value"=w297) -> ()  [unwired: 2 in, 2 out]
                n256 = Close File(refnum=w291, error in=w300) -> (error out=w290:errorcluster)  [unwired: 1 out]
                n257 = call "Option to string.vi"("String in"=w283) -> ("String out"=w282:string)  [unwired: 10 in]
                n258 = call "Option to string.vi"("String in"=w285) -> ("String out"=w284:string)  [unwired: 10 in]
                n259 = call <vilib>:"Space Constant.vi"() -> ("String"=w288:string)
                n260 = call <vilib>:"Simple Error Handler.vi"("error in (no error)"=w290) -> ()  [unwired: 4 in, 5 out]
                n261 = property on="COM Port" class="VISAName"("Text.Text"=w284) -> ()  [unwired: 2 in, 2 out]
                n262 = Search and Replace String(replace all?=TRUE ("replace all? (F)"), input string=w282, search string=">", replace string=w288) -> (result string=w287:string)  [unwired: 4 in, 3 out]
                n263 = property on="Data input file" class="Path"("Text.Text"=w287) -> ()  [unwired: 2 in, 2 out]
              }
            }
          }
        }
      }
      event "Reset everything": Value Change {
        n264 = event-data() -> ()  [unwired: 1 in, 6 out]
        n265 = Two Button Dialog(message="Are you sure you want to completely reset all program data and stop communication? You will have to recalibrate frequencies, and the current automatic seek mode state will be forgotten. Additionally, this will not move the motor back to a known position, so if you restart the motor after doing this, all saved frequency calibrations will be invalidated.", 1:"Nah, nevermind" ("F button name (\"Cancel\")"), 2:"DO IT" ("T button name (\"OK\")")) -> (T button?=w304:bool)
        n266 = case shown="True" w304 {
          tunnel: w308 -> [_ w309]
          frame False {
          }
          frame True {
            n267 = flat-sequence {
              tunnel: w309 -> [w311]
              frame #0 {
                n268 = control-ref of="This VI"() -> (w310:refnum<vi>)
                n269 = invoke class="VI" method="Default Vals.Reinit All"(reference=w310) -> ()  [unwired: 2 in, 3 out]
              }
              frame #1 {
                n270 = call "Signal.vi"("Signaller in"=w311) -> ()  [unwired: 9 in, 2 out]
              }
            }
          }
        }
      }
      event "Stop communication": Value Change {
        # "Move motor back to a known position (position 0)"
        n271 = event-data() -> ()  [unwired: 1 in, 5 out]
        n272 = property on="Motor position (rev)" class="DigNum (strict)"() -> ("Value"=w315:dbl)  [unwired: 2 in, 2 out]
        n273 = Negate(x=w315) -> (-x=w314:dbl)
        n274 = call-dynamic "Move.vi"("Amount (rev)"=w314, "Motor in"=w313) -> ("error out"=w312:errorcluster)  [unwired: 8 in, 1 out]
        n275 = call "Signal.vi"("error in (no error)"=w312, "Signaller in"=w316) -> ()  [unwired: 8 in, 2 out]
      }
      event Timeout {
        n276 = event-data() -> ()  [unwired: 1 in, 2 out]
      }
    }
  }
  n277 = while {
    tunnel: w12 -> [w319]
    shift-right: [w324] -> _
    shift-left: w19 -> [w328]
    shift-right: [w326] -> _
    shift-left: w18 -> [w327]
    tunnel: w3 -> [w325]
    shift-right: [w317] -> _
    shift-left: w13 -> [w318]
    stop <- w332 stop-if-true
    n278 = call "Peek or default.vi"("Signaller in"=w319) -> ("Has signal?"=w332:bool)  [unwired: 8 in, 2 out]
    n279 = property on="Automatic mode on/off" class="Bool (strict)"() -> ("Value"=w323:bool)  [unwired: 2 in, 2 out]
    n280 = case shown="True" w323 {
      tunnel: "Data input file" -> [w334 w337]
      tunnel: [w334 w335] -> w321
      tunnel: [FALSE ("Filepath valid?") w336] -> w320
      frame False {
      }
      frame True {
        # "Prompt the user for a data filepath if none is selected"
        n281 = call "Select filepath if none.vi"("Error message"="Must select a data file to use automatic mode.", "Selector prompt"="Select a data file", "Filepath in"=w337) -> ("Filepath valid?"=w336:bool, "Filepath out"=w335:path)
        n282 = case shown="True" w336 {
          tunnel: w335 -> [_ w341]
          frame False {
            # "Turn off automatic mode so the user isn't\nprompted again and again"
            n283 = property on="Automatic mode on/off" class="Bool (strict)"("Val(Sgnl)"=FALSE ("Value (Signaling)")) -> ()  [unwired: 2 in, 2 out]
          }
          frame True {
            # "Update the filepath control to this\nnewly selected path"
            n284 = property on="Data input file" class="Path"("Value"=w341) -> ()  [unwired: 2 in, 2 out]
          }
        }
      }
    }
    n285 = property on="Alarm" class="Bool (strict)"() -> ("Value"=w331:bool)  [unwired: 2 in, 2 out]
    n286 = Not(x=w331) -> (.not. x?=w330:bool)
    n287 = And(x=w320, y=w330) -> (x .and. y?=w329:bool)
    n288 = case shown="True" w329 {
      tunnel: [w344 w360] -> w324
      tunnel: w328 -> [w344 w359]
      tunnel: w327 -> [w343 w358]
      tunnel: [w343 w357] -> w326
      tunnel: w325 -> [_ w356]
      tunnel: w321 -> [_ w354]
      tunnel: w319 -> [_ w353]
      tunnel: w318 -> [w342 w352]
      tunnel: [w342 w345] -> w317
      frame False {
      }
      frame True {
        w355 = u32 1000  # ms to wait between samples
        n289 = call "Get last row.vi"("Data input file"=w354) -> ("last row"=w351:string[])
        n290 = call "Input data row.vi"("Last row of data file"=w351, "Automatic Mode in"=w352) -> ("Automatic Mode out"=w350:refnum<class "Automatic Mode.lvclass">)  [unwired: 8 in, 1 out]
        n291 = call "Get number of samples taken.vi"("Automatic Mode in"=w350) -> ("Number of samples taken"=w349:i32, "Automatic Mode out"=w348:refnum<class "Automatic Mode.lvclass">)  [unwired: 8 in, 1 out]
        n292 = call "Has all samples.vi"("Automatic Mode in"=w348) -> ("Has all samples?"=w347:bool, "Automatic Mode out"=w346:refnum<class "Automatic Mode.lvclass">)  [unwired: 8 in, 1 out]
        n293 = property on="Samples taken" class="DigNum (strict)"("Value"=w349) -> ()  [unwired: 2 in, 2 out]
        n294 = Wait Until Next ms Multiple(millisecond multiple=w355) -> ()  [unwired: 1 out]
        n295 = case shown="True" w347 {
          tunnel: [w363 w375] -> w360
          tunnel: w359 -> [w363 w384]
          tunnel: w358 -> [w362 w387]
          tunnel: [w362 w365] -> w357
          tunnel: w356 -> [_ w386]
          tunnel: w353 -> [_ w380]
          tunnel: w346 -> [w361 w379]
          tunnel: [w361 w374] -> w345
          frame False {
          }
          frame True {
            w381 = 5  # Seconds to wait
            w373 = 0  # Reset array pos to 0
            # "Move in the appropriate direction\n(true means \"move up\") using the\nappropriate distance; the direction\nand distance are determined by the\nresults of the previous conditional\ncomparing the old and new rates"
            # "Change directions if the rate at this position\nisn't at least as good as the last one"
            # "If we're seeking positive, we\nwant the new rate to be at least\nas large as the last one; if we're\nseeking negative, it's the opposite"
            # "Give the motor some time;\nusing \"wait no block\" instead\nof the built-in delay function\nmakes it so that we can stop\nthe VI while it's waiting and not\nhave to wait the full 5 seconds before\nit shuts down"
            n296 = call "Get last data point.vi"("Automatic Mode in"=w379) -> ("Polarization"=w377:dbl, "Eventnum"=w378:i64, "Automatic Mode out"=w376:refnum<class "Automatic Mode.lvclass">)  [unwired: 7 in, 1 out]
            n297 = call "Calculate average rate.vi"("Automatic Mode in"=w376) -> ("Average rate"=w375:dbl, "Automatic Mode out"=w374:refnum<class "Automatic Mode.lvclass">)  [unwired: 8 in, 1 out]
            n298 = flat-sequence {
              tunnel: w377 -> [w396]
              tunnel: w375 -> [w397]
              tunnel: w378 -> [w398]
              frame #0 {
                # "Update the data points on the front panel"
                "Polarization" <- w396
                "Rate" <- w397
              }
              frame #1 {
                # "The eventnum must be updated last to maintain\ncompatibility with the grapher, which expects\nit to be the last value updated"
                "Eventnum" <- w398
              }
            }
            n299 = case shown="True" "Seek positive polarization" {
              tunnel: w384 -> [w391 w395]
              tunnel: [w390 w394] -> w383
              tunnel: w375 -> [w392 w393]
              frame False {
                n300 = Less Or Equal?(x=w392, y=w391) -> (x <= y?=w390:bool)
              }
              frame True {
                n301 = Greater Or Equal?(x=w393, y=w395) -> (x >= y?=w394:bool)
              }
            }
            n302 = case shown="False" w383 {
              tunnel: w387 -> [w413 w419]
              tunnel: [w412 w419] -> w366
              tunnel: "Step size (rev)" -> [w409 w418]
              tunnel: [w408 w418] -> w385
              frame False {
                w411 = 0.001  # Minimum step size
                # "Change directions and adjust step size"
                n303 = Greater?(x=w409, y=w411) -> (0:w410:bool)
                n304 = case shown="True" w410 {
                  tunnel: w409 -> [w414 w416]
                  tunnel: [w414 w415] -> w408
                  frame False {
                  }
                  frame True {
                    w417 = 0.9  # Step size diminuation factor
                    n305 = Multiply(x=w416, y=w417) -> (x*y=w415:dbl)
                  }
                }
                n306 = Not(x=w413) -> (.not. x?=w412:bool)
                n307 = property on="Step size (rev)" class="DigNum (strict)"("Value"=w408) -> ()  [unwired: 2 in, 2 out]
              }
              frame True {
              }
            }
            n308 = case shown="True" "Seek positive polarization" {
              tunnel: ["Negative seek bounds" "Positive seek bounds"] -> w368
              frame False {
              }
              frame True {
              }
            }
            n309 = case shown="True" w366 {
              tunnel: w386 -> [w403 w406]
              tunnel: w385 -> [w402 w407]
              tunnel: [w400 w404] -> w371
              tunnel: [w399 w405] -> w370
              frame False {
                n310 = Negate(x=w402) -> (-x=w401:dbl)
                n311 = call-dynamic "Move.vi"("Amount (rev)"=w401, "Motor in"=w403) -> ("error out"=w399:errorcluster, "Motor out"=w400:refnum<class "Motor.lvclass">)  [unwired: 8 in]
              }
              frame True {
                n312 = call-dynamic "Move.vi"("Amount (rev)"=w407, "Motor in"=w406) -> ("error out"=w405:errorcluster, "Motor out"=w404:refnum<class "Motor.lvclass">)  [unwired: 8 in]
              }
            }
            n313 = property on="Fit parameters" class="Clust (strict)"() -> ("Value"=w364:cluster{"Slope":dbl, "Intercept":dbl})  [unwired: 2 in, 2 out]
            n314 = call-dynamic "Move to bounds.vi"("error in (no error)"=w370, "Fit parameters"=w364, "Seek bounds"=w368, "Motor in"=w371) -> ("error out"=w369:errorcluster, "Was outside?"=w367:bool)  [unwired: 5 in, 1 out]
            n315 = Exclusive Or(1:w367, 2:w366) -> (0:w365:bool)
            n316 = call "Wait on signal.vi"("error in (no error)"=w369, "Seconds to wait"=w381, "Signaller in"=w380) -> ()  [unwired: 7 in, 2 out]
            "Samples taken" <- w373
          }
        }
      }
    }
  }
  n317 = case shown="True" w8 {
    frame False {
    }
    frame True {
      n318 = call "Display Message to User2"() -> ("Thanks, I'll try that"=w420:bool)  [unwired: 10 in, 1 out]
      n319 = Stop(stop? (T)=w420) -> ()
    }
  }
  n320 = call-dynamic "Destroy.vi"("Motor in"=w1) -> ()  [unwired: 10 in, 1 out]
  n321 = call "Destroy.vi"("Signaller in"=w20) -> ("error out"=w17:errorcluster)  [unwired: 10 in]
  n322 = flat-sequence {
    tunnel: w17 -> [_]
    frame #0 {
      # "Turn automatic mode off when the VI is stopped;\nthat way, it doesn't try to start in automatic\nmode immediately on the next startup"
      n323 = property on="Automatic mode on/off" class="Bool (strict)"("Val(Sgnl)"=FALSE ("Automatic mode on/off")) -> ()  [unwired: 2 in, 2 out]
    }
  }
